vi "GetWlRaw.vi"(8 "error in (no error)":errorcluster, 10 "Integration Time":i32, 11 "SpectRef In":T1) -> (0 "error out":errorcluster, 1 "SpectRef Out":T1, 2 "SpectrumSplit":dbl[](array[numeric]), 3 "WavelengthSplit":dbl[](array[numeric]), 4 "Saturated?":bool, 5 "MaxSpectrum":dbl, 7 "delta":dbl)   [LabVIEW 2012]
uses:
  Controls/USB4000_Data.ctl
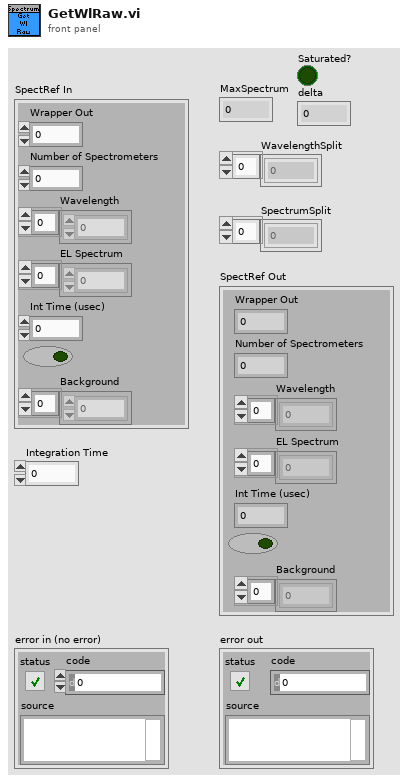
[diagram p1: front panel]
types:
  T1 = typedef "USB4000_Data.ctl" = cluster{"Wrapper Out":u32, "Number of Spectrometers":i32, "Wavelength":dbl[], "EL Spectrum":dbl[], "Int Time (usec)":i32, bool, "Background":dbl[]}
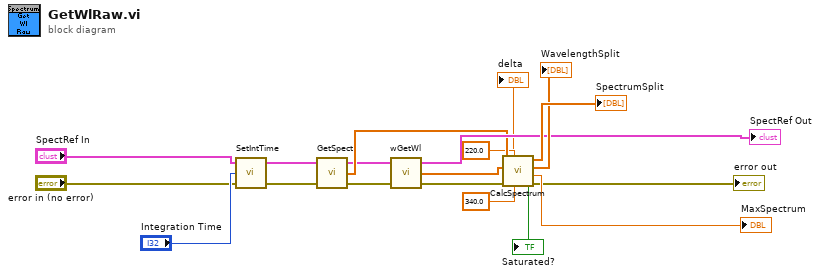
[diagram p0: block diagram]
diagram:
  n1 = call "SetIntTime.vi"("error in"="error in (no error)", "Integration Time"="Integration Time", "SpectRef In"="SpectRef In") -> ("error out"=w5:errorcluster, "SpectRef Out"=w3:T1)  [unwired: 1 in]
  n2 = call "GetSpect.vi"("error in (no error)"=w5, "SpectRef In"=w3) -> ("error out"=w6:errorcluster, "Spectrum Values"=w12:dbl[], "SpectRef Out"=w4:T1)  [unwired: 1 in]
  n3 = call "wGetWl.vi"("error in (no error)"=w6, "SpectRef In"=w4) -> ("error out"=w14:errorcluster, "WL Values"=w13:dbl[], "SpectRef Out"=→"SpectRef Out":T1)  [unwired: 1 in]
  n4 = call "CalcSpectrum.vi"("WlStop"=340.0, "WlStart"=220.0, "error in (no error)"=w14, "Wavelength"=w13, "Spectrum"=w12) -> ("error out"=→"error out":errorcluster, "MaxSpectrum"=→"MaxSpectrum":dbl, "WavelengthSplit"=→"WavelengthSplit":dbl[], "SpectrumSplit"=→"SpectrumSplit":dbl[], "Saturated?"=→"Saturated?":bool, "delta"=→"delta":dbl)  [unwired: 1 in]
